vi "Write Delimited Spreadsheet (string).vi"(0 "Path":path, 1 "format string":string, 5 "2D data":string[][](array[string]), 7 "1D data":string[](array[string]), 9 "append to file?":bool, 11 "error in":errorcluster, 12 "transpose? (no:F)":bool, 13 "delimiter (\\t)":string) -> (4 "path":path, 15 "error out":errorcluster)   [LabVIEW 2018]
panel:
  in  "prompt":string
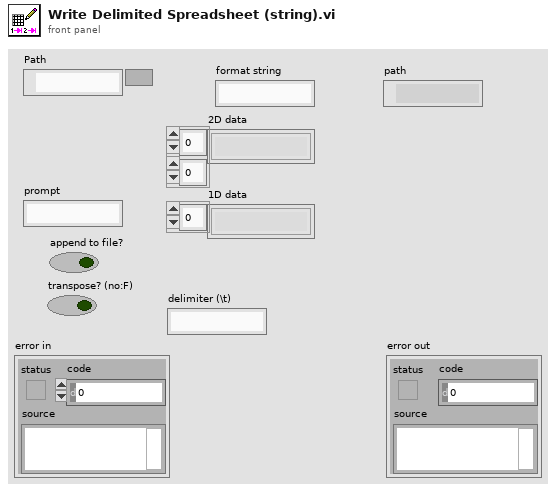
[diagram p1: front panel]
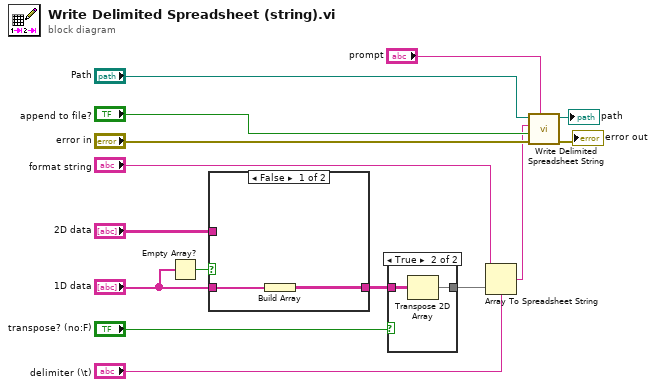
[diagram p0: block diagram]
diagram:
  n1 = Empty Array?(array="1D data") -> (empty?=w11:bool)
  n2 = case shown="False" w11 {
    tunnel: "1D data" -> [w17 _]
    tunnel: "2D data" -> [_ w18]
    tunnel: [w16 w18] -> w8
    frame False {
      n3 = Build Array(w17) -> (w16:string[][])
    }
    frame True {
    }
  }
  n4 = case shown="True" "transpose? (no:F)" {
    tunnel: w8 -> [w19 w21]
    tunnel: [w19 w20] -> w6
    frame False {
    }
    frame True {
      n5 = Transpose 2D Array(2D array=w21) -> (transposed array=w20:string[][])
    }
  }
  n6 = Array To Spreadsheet String(delimiter (Tab)="delimiter (\\t)", array=w6, 3:"format string") -> (spreadsheet string=w3:string)
  n7 = call "Write Delimited Spreadsheet String.vi"("prompt"="prompt", "error in"="error in", "append to file?"="append to file?", "spreadsheet string"=w3, "Path"="Path") -> ("error out"=→"error out":errorcluster, "path"=→"path":path)  [unwired: 5 in]
